vi "Dismantle Filename.vi"(4 "error in (no error)":errorcluster, 7 "file":path) -> (0 "error out":errorcluster, 1 "lowercase file extension":string, 2 "file name without extension":string, 3 "stripped path":path)   [LabVIEW 2014]
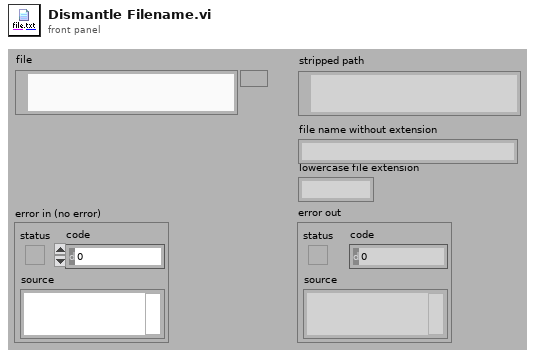
[diagram p1: front panel]
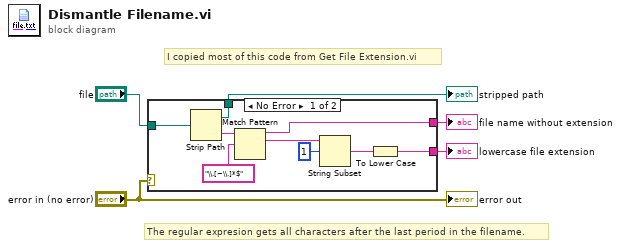
[diagram p0: block diagram]
diagram:
  # "I copied most of this code from Get File Extension.vi"
  # "The regular expresion gets all characters after the last period in the filename."
  n1 = case shown="No Error" "error in (no error)" {
    tunnel: "file" -> [w13 _]
    tunnel: [w11 _] -> w4
    tunnel: [w7 _] -> w3
    tunnel: [w6 _] -> w1
    frame No Error {
      n2 = Strip Path(path=w13) -> (stripped path=w6:path, name=w12:string)
      n3 = Match Pattern(string=w12, regular expression="\\.[~\\.]*$") -> (before substring=w7:string, match substring=w14:string)  [unwired: 1 in, 2 out]
      n4 = String Subset(string=w14, offset (0)=1) -> (substring=w10:string)  [unwired: 1 in]
      n5 = To Lower Case(string=w10) -> (all lower case string=w11:string)
    }
    frame Error {
    }
  }
  "stripped path" <- w1
  "lowercase file extension" <- w4
  "file name without extension" <- w3
  "error out" <- "error in (no error)"
